vi "PingTest.vi"(10 "Channel Name":string, 11 "IP Address":string) -> (2 "Comment":string, 3 "Reading":dbl format="%.3f")   [LabVIEW 2015]
panel:
  out "concatenated string":string
  out "standard error":string
  out "standard output":string
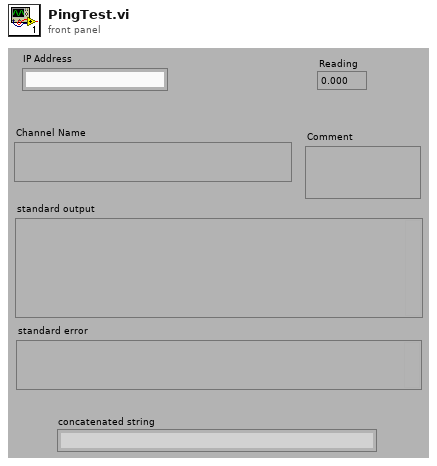
[diagram p1: front panel]
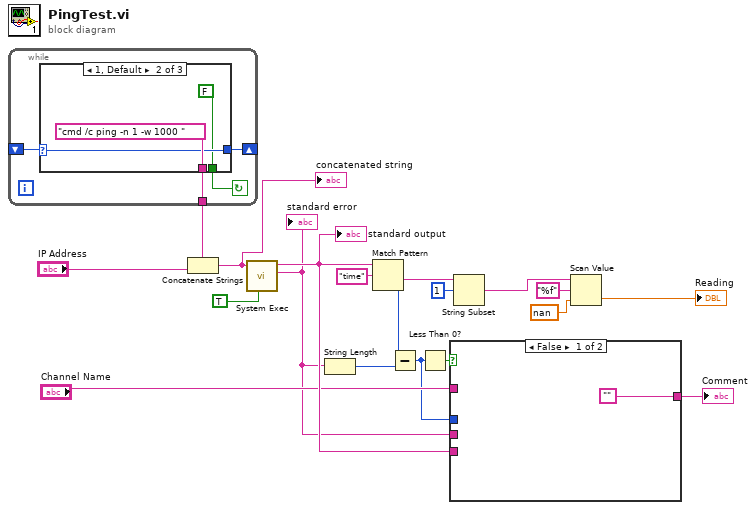
[diagram p0: block diagram]
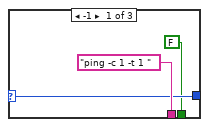
[diagram p2: hidden frame]
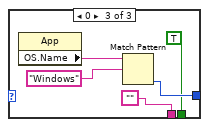
[diagram p3: hidden frame]
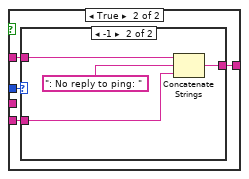
[diagram p4: hidden frame]
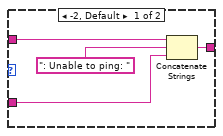
[diagram p5: hidden frame]
diagram:
  n1 = while {
    shift-right: [w22] -> _
    shift-left: _ -> [w23]
    tunnel: [w21] -> w5
    stop <- w20 continue-if-true
    n2 = case shown="1, Default" w23 {
      selector: w23 -> [w25 w28 _]
      tunnel: [w25 w28 w32] -> w22
      tunnel: ["ping -c 1 -t 1 " ("string") "cmd /c ping -n 1 -w 1000 " ("string") ""] -> w21
      tunnel: [FALSE FALSE TRUE] -> w20
      frame -1 {
      }
      frame 1, Default {
      }
      frame 0 {
        n3 = property class="App"() -> ("OS.Name"=w34:string)  [unwired: 2 in, 2 out]
        n4 = Match Pattern(string=w34, regular expression="Windows") -> (offset past match=w32:i32)  [unwired: 4 out]
      }
    }
  }
  n5 = Concatenate Strings(w5, "IP Address") -> (w19:string)
  "concatenated string" <- w19
  n6 = call <vilib>:"System Exec.vi"("run minimized? (F)"=TRUE, "command line"=w19) -> ("standard error"=w8:string, "standard output"=w12:string)  [unwired: 4 in, 4 out]
  "standard output" <- w12
  "standard error" <- w8
  n7 = String Length(string=w8) -> (length=w11:i32)
  n8 = Match Pattern(string=w12, regular expression="time") -> (after substring=w17:string, offset past match=w10:i32)  [unwired: 3 out]
  n9 = Subtract(x=w10, y=w11) -> (x-y=w6:i32)
  n10 = Less Than 0?(x=w6) -> (x < 0?=w7:bool)
  n11 = case shown="False" w7 {
    tunnel: w12 -> [_ w39]
    tunnel: ["" w38] -> w13
    tunnel: "Channel Name" -> [_ w37]
    tunnel: w8 -> [_ _]
    tunnel: w6 -> [_ w36]
    frame False {
    }
    frame True {
      n12 = case shown="-1" w36 {
        tunnel: w39 -> [w41 w46]
        tunnel: [w40 w45] -> w38
        tunnel: w37 -> [w42 w44]
        frame -2, Default {
          n13 = Concatenate Strings(w42, ": Unable to ping: " ("string"), w41) -> (w40:string)
        }
        frame -1 {
          n14 = Concatenate Strings(w44, ": No reply to ping: " ("string"), w46) -> (w45:string)
        }
      }
    }
  }
  "Comment" <- w13
  n15 = String Subset(string=w17, offset (0)=1) -> (substring=w4:string)  [unwired: 1 out]
  n16 = Scan Value(string=w4, format string="%f", default (0 dbl)=nan) -> (value=→"Reading":dbl)  [unwired: 1 out]
